vi "MouvementDirection.vi"(3 "Increment corrected for direction":i16) -> (0 "Sign of corrected target":bool, 1 "Mouvement Direction":i16)   [LabVIEW 2016]
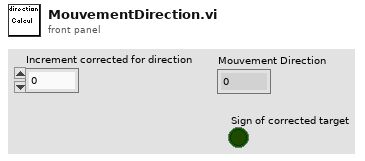
[diagram p1: front panel]
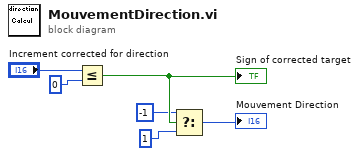
[diagram p0: block diagram]
diagram:
  n1 = Less Or Equal?(x="Increment corrected for direction", y=i16 0) -> (x <= y?=w5:bool)
  "Sign of corrected target" <- w5
  n2 = Select(t=i16 -1, s=w5, f=i16 1) -> (s? t:f=→"Mouvement Direction":i16)
